vi "Named_Serial_Comms_orig.vi"(0 "Channel Name":string, 1 "Write String":string, 2 "Timeout/ms":u32=500, 4 "!Error retries":i32=10, 6 "!Timeout retries":i32=3, 9 "Port Name":string, 11 "Term Grep":string="\r$", 12 "Log Errors?":bool=TRUE, 13 "Terminate Count":i32) -> (3 "Read":string="This is simulation mode", 10 "millisecond timer value":u32, 14 "Timed out":bool, 15 "Serial Error":bool)   [LabVIEW 2010]
doc: "The Serial Communication VI performs bidirectional communication with a port. It initializes the port, writes a string to the port, and performs a read with timeout. The Read with Timeout will wait until a terminating character is received or the time limit is up, whichever comes first.\nThe initialisation parameters, terminating character, and timeout, are all set in the Serial Setup Global."
uses:
  Port_Params.ctl
  <vilib>/Instr/serial.llb/serpConfig.vi
panel:
  out "Buffer Trash":string
  out "Check Loops":i32
  out "Time Start":u32
  out "byte count":u32
  out "Terminated?":bool
  out "Case":string="Simulate"
  out "!Error retries remaining":i32=10
  out "length":i32
  out "Read chunks":string[](array[string])
  in  "Force setup reload":bool
  out "Port Initialised?":bool[](array[boolean])
  out "load setups error":bool
  out "Setting Number":i32
  in  "Error Description":string
  out "Read Loops":i32
  out "Audit trail":string[](array[string])=["Start", "Simulate"]
  in  "Save Setups?":bool
  out "Close Port error":i32
  out "read error code":i32
  out "n-bytes error code":i32
  out "Ports having file settings":string[](array[string])
  in  "Uppercase?":bool
  in  "Append Return?":bool
  out "Write error":i32
  in  "!stop":bool
  out "Port Initialisation Parameters":T1={"Name"="", "flow control etc."={"input XON/XOFF"=FALSE, "input HW Handshake"=FALSE, "input alt HW HShk"=FALSE, "output XON/XOFF"=FALSE, "output HW Handshake"=FALSE, "output alt HW HShk"=FALSE, "XOFF byte "=0, "XON byte"=0, "parity err byte"=0}, "buffer size"=0, "baud rate"=9600, "data bits"=8, "stop bits"=enum."1 bit", "parity"=enum."no parity"} {"flow control etc."."parity err byte" format="%.0x"; "flow control etc."."XON byte" format="%.0x"; "flow control etc."."XOFF byte" format="%.0x"; "data bits" min=5 max=8 step=1}
  out "Port Number":i32
  out "Initialise error":i32
  out "enumerated ports":string[](array[string])
  in  "Port Settings Array":T1[](array[typedef]) {"flow control etc."."parity err byte" format="%.0x"; "flow control etc."."XON byte" format="%.0x"; "flow control etc."."XOFF byte" format="%.0x"; "data bits" min=5 max=8 step=1}
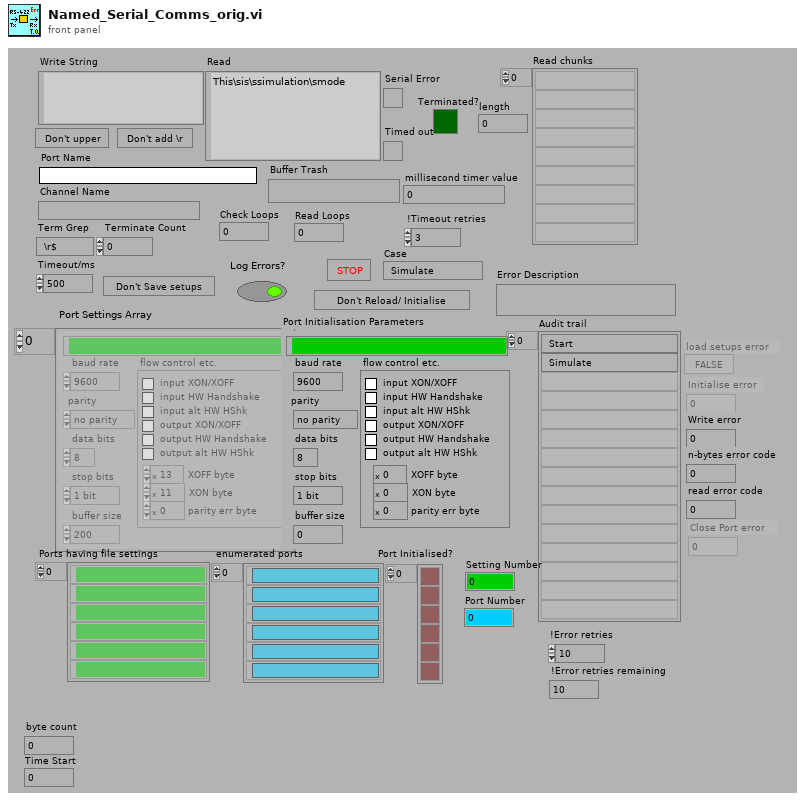
[diagram p1: front panel]
types:
  T1 = typedef "Port_Params.ctl" = cluster{"Name":string, "flow control etc.":cluster{"input XON/XOFF":bool, "input HW Handshake":bool, "input alt HW HShk":bool, "output XON/XOFF":bool, "output HW Handshake":bool, "output alt HW HShk":bool, "XOFF byte ":u8, "XON byte":u8, "parity err byte":u16}, "buffer size":u16, "baud rate":u32, "data bits":u16, "stop bits":enum16{"1 bit", "1.5 bits", "2 bits"}, "parity":enum16{"no parity", "odd parity", "even parity", "mark parity", "space parity"}}
  T2 = cluster{"input XON/XOFF":bool, "input HW Handshake":bool, "input alt HW HShk":bool, "output XON/XOFF":bool, "output HW Handshake":bool, "output alt HW HShk":bool, "XOFF byte ":u8, "XON byte":u8, "parity err byte":u16}
  T3 = enum16{"no parity", "odd parity", "even parity", "mark parity", "space parity"}
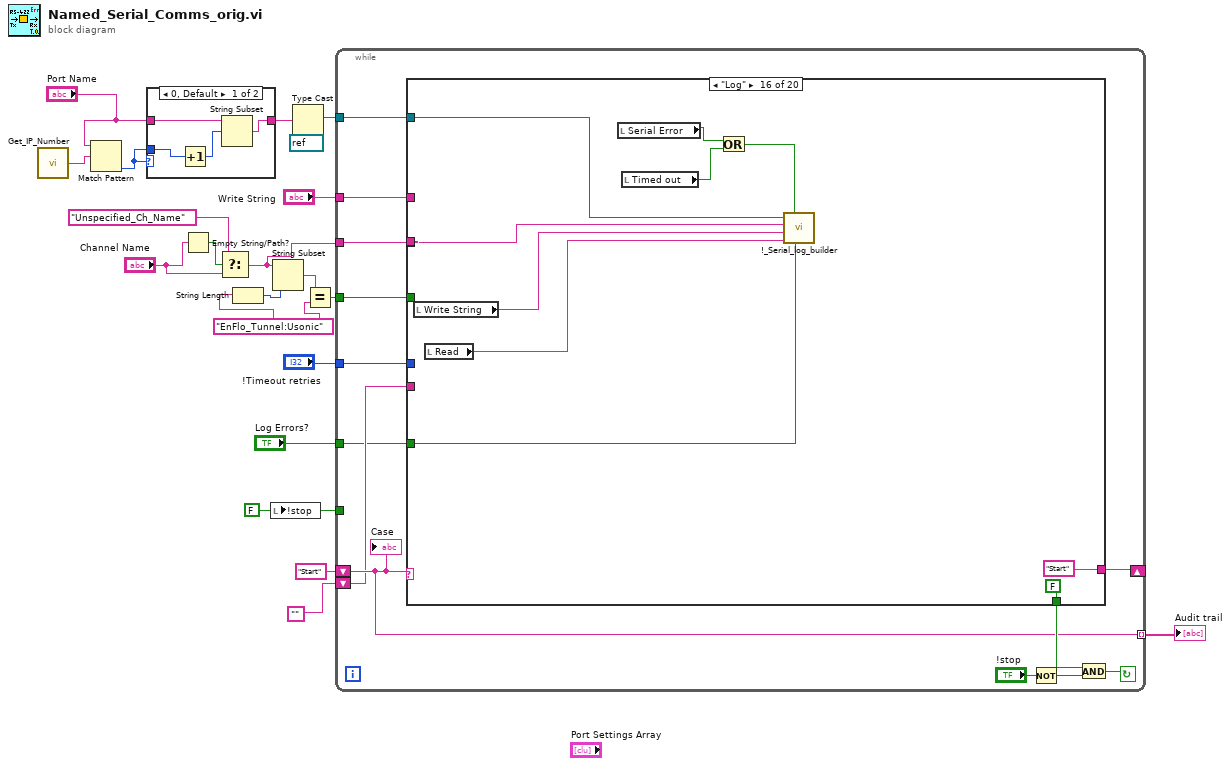
[diagram p0: block diagram]
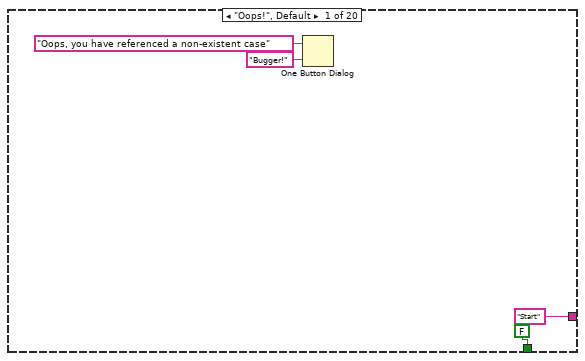
[diagram p3: hidden frame]
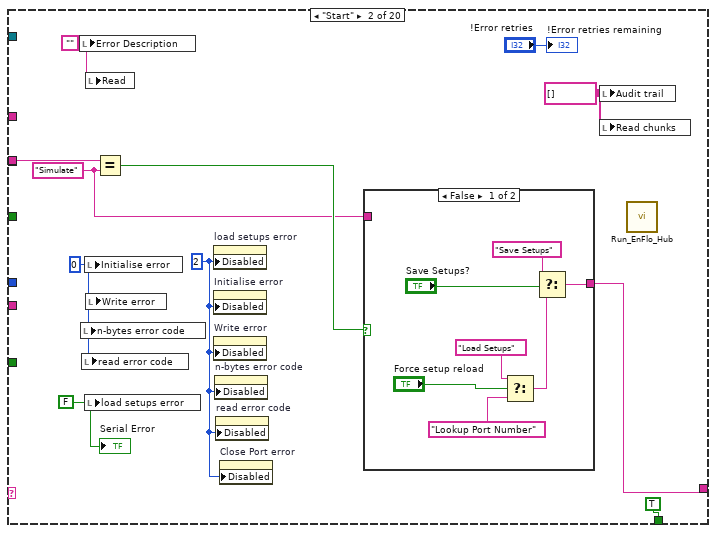
[diagram p4: hidden frame]
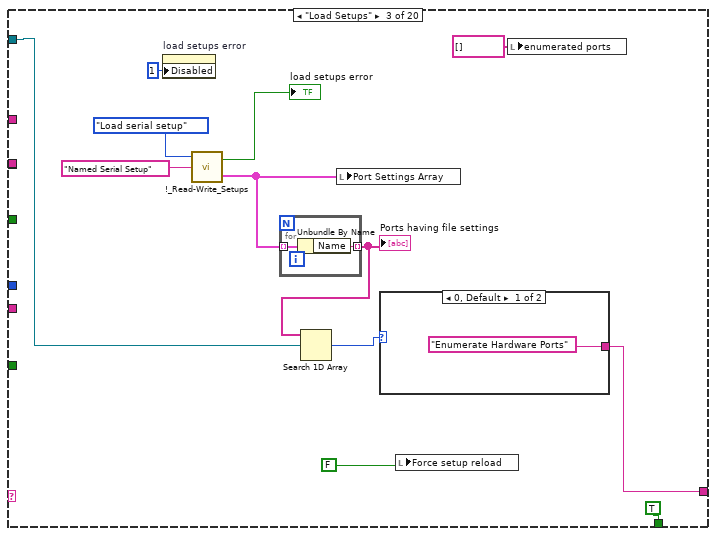
[diagram p6: hidden frame]
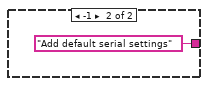
[diagram p7: hidden frame]
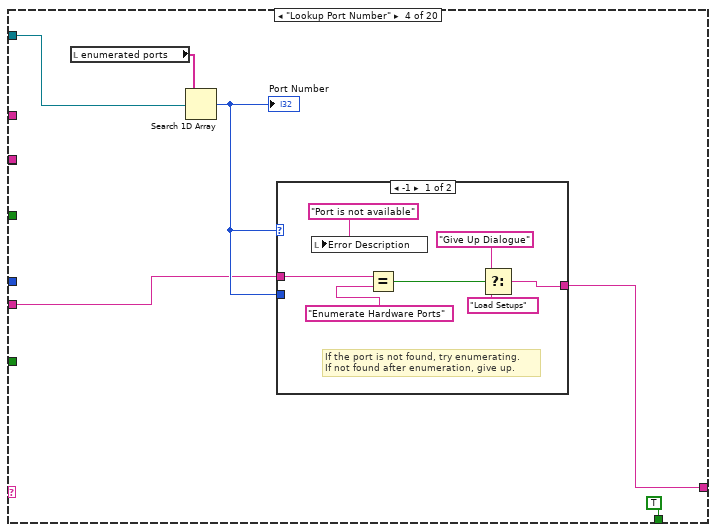
[diagram p8: hidden frame]
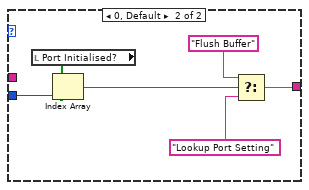
[diagram p9: hidden frame]
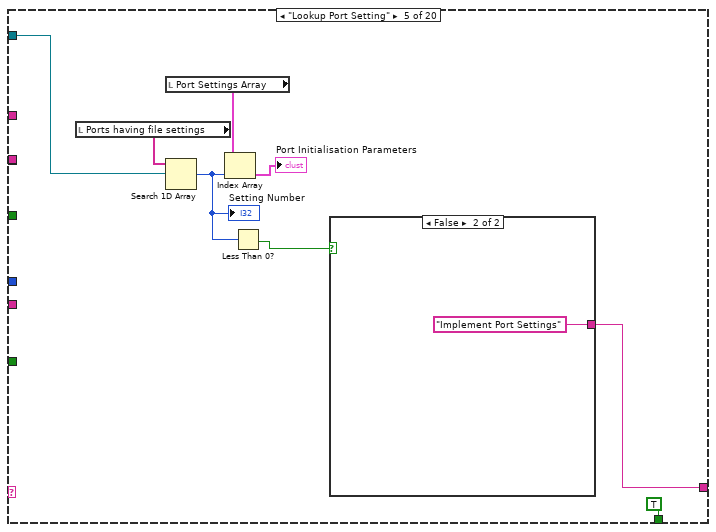
[diagram p10: hidden frame]
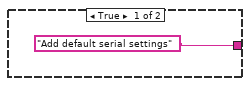
[diagram p11: hidden frame]
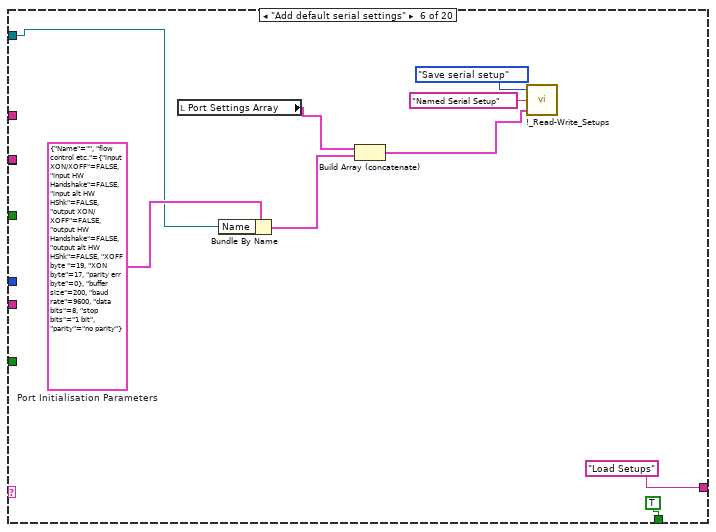
[diagram p12: hidden frame]
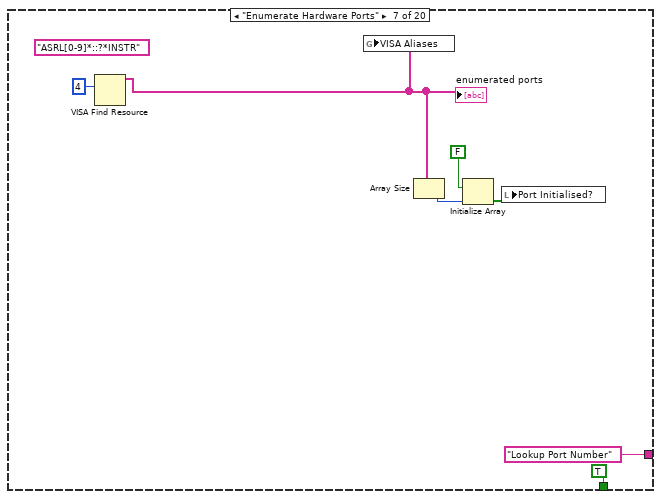
[diagram p13: hidden frame]
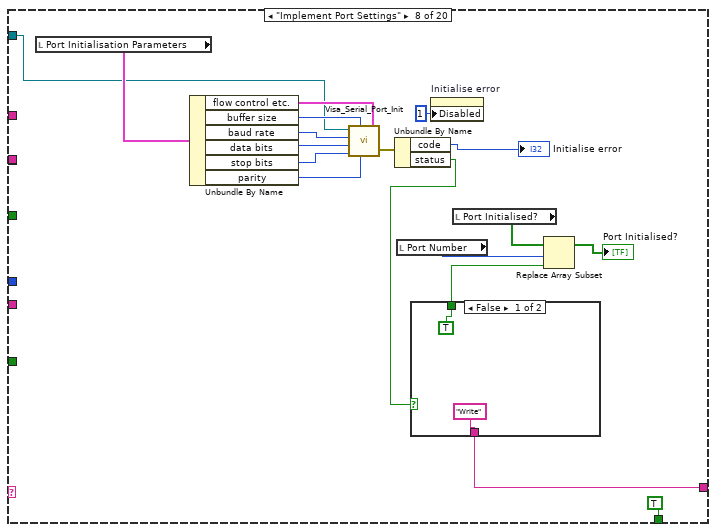
[diagram p14: hidden frame]
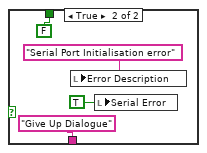
[diagram p15: hidden frame]
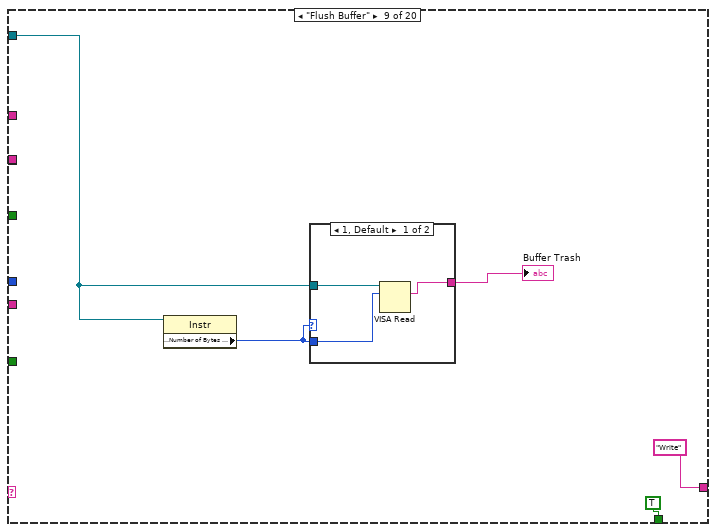
[diagram p16: hidden frame]
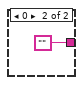
[diagram p17: hidden frame]
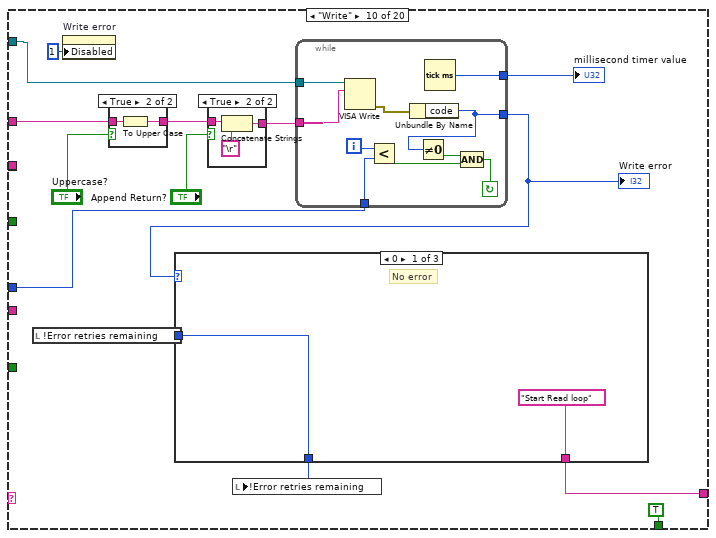
[diagram p18: hidden frame]
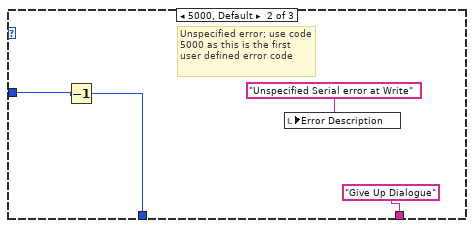
[diagram p19: hidden frame]
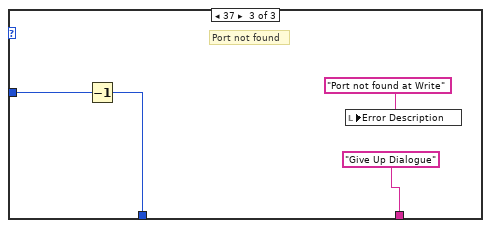
[diagram p20: hidden frame]
diagram:
  w13 = "EnFlo_Tunnel:Usonic"
  w19 = FALSE ("!stop")
  n1 = call "Get_IP_Number.vi"() -> ("IP Number"=w8:string)
  n2 = Match Pattern(string="Port Name", regular expression=w8) -> (offset past match=w9:i32)  [unwired: 1 in, 3 out]
  n3 = case shown="0, Default" w9 {
    tunnel: [w22 w26] -> w6
    tunnel: "Port Name" -> [w23 w26]
    tunnel: w9 -> [w25 _]
    frame 0, Default {
      n4 = Increment(x=w25) -> (x+1=w24:i32)
      n5 = String Subset(string=w23, offset (0)=w24) -> (substring=w22:string)  [unwired: 1 in]
    }
    frame -1 {
    }
  }
  n6 = Empty String/Path?(string/path="Channel Name") -> (empty?=w4:bool)
  n7 = Select(t="Unspecified_Ch_Name", s=w4, f="Channel Name") -> (s? t:f=w3:string)
  n8 = String Length(string=w13) -> (length=w15:i32)
  n9 = local write "!stop"(w19) -> ()
  n10 = String Subset(string=w3, length (rest)=w15) -> (substring=w14:string)  [unwired: 1 in]
  n11 = Type Cast(type=refnum<visa-resource-name> refnum ("dup VISA resource name"), x=w6) -> (*(type *) &x=w11:refnum<visa-resource-name>)
  n12 = Equal?(x=w14, y=w13) -> (x = y?=w12:bool)
  n13 = while {
    tunnel: "!Timeout retries" -> [w29]
    tunnel: w3 -> [w31]
    shift-left: "" -> [w30]
    tunnel: [w32] -> w18 mode=indexing
    tunnel: w19 -> [_]
    shift-left: "Start" -> [w32]
    shift-right: [w33] -> _
    tunnel: "Write String" -> [w38]
    tunnel: w11 -> [w39]
    tunnel: w12 -> [w28]
    tunnel: "Log Errors?" -> [w27]
    stop <- w36 continue-if-true
    n14 = case shown="\"Log\"" w32 {
      tunnel: w39 -> [_ _ w64 w84 w104 w113 _ w127 w148 w157 _ w208 w236 _ _ w300 w310 _ w332 _]
      tunnel: w38 -> [_ _ _ _ _ _ _ _ _ w166 _ _ _ _ _ _ w313 _ _ _]
      tunnel: ["Start" ("f") w54 w67 w81 w100 "Load Setups" ("f") "Lookup Port Number" w132 "Write" ("f") w162 "Bytes At Serial Port?" ("f") w213 w250 w265 w295 "Start" "Start" "Start" "Start" ("f") "Load Setups" ("f")] -> w33
      tunnel: [FALSE TRUE TRUE TRUE TRUE TRUE TRUE TRUE TRUE TRUE TRUE TRUE TRUE TRUE TRUE FALSE FALSE TRUE FALSE TRUE] -> w37
      tunnel: w31 -> [_ w47 _ _ _ _ _ _ _ _ _ _ _ _ _ w306 _ _ _ _]
      tunnel: w31 -> [_ _ _ _ _ _ _ _ _ _ _ _ _ _ _ _ w311 _ _ _]
      tunnel: w30 -> [_ _ _ w79 _ _ _ _ _ _ _ _ _ _ _ _ _ _ _ _]
      tunnel: w29 -> [_ _ _ _ _ _ _ _ _ w158 _ w210 _ _ _ _ _ _ _ _]
      tunnel: w28 -> [_ _ _ _ _ _ _ _ _ _ _ _ w240 _ _ _ _ _ _ _]
      tunnel: w27 -> [_ _ _ _ _ _ _ _ _ _ _ _ _ _ _ w299 _ _ _ _]
      frame "Oops!", Default {
        n15 = One Button Dialog(message="Oops, you have referenced a non-existent case", button name ("OK")="Bugger!") -> ()  [unwired: 1 out]
      }
      frame "Start" {
        w44 = string[] [] ("Audit trail")
        w45 = "Simulate" ("y")
        w51 = 0 ("Initialise error")
        w49 = FALSE
        w50 = u8 2 ("Write Attribute")
        w52 = ""
        n16 = local write "Error Description"(w52) -> ()
        n17 = local write "n-bytes error code"(w51) -> ()
        n18 = local write "read error code"(w51) -> ()
        n19 = local write "Initialise error"(w51) -> ()
        n20 = local write "load setups error"(w49) -> ()
        n21 = local write "Read"(w52) -> ()
        n22 = local write "Write error"(w51) -> ()
        n23 = Equal?(x=w47, y=w45) -> (x = y?=w46:bool)
        n24 = property on="load setups error" class="Bool (strict)"("Disabled"=w50) -> ()  [unwired: 2 in, 2 out]
        n25 = property on="Initialise error" class="DigNum (strict)"("Disabled"=w50) -> ()  [unwired: 2 in, 2 out]
        n26 = property on="Write error" class="DigNum (strict)"("Disabled"=w50) -> ()  [unwired: 2 in, 2 out]
        n27 = property on="n-bytes error code" class="DigNum (strict)"("Disabled"=w50) -> ()  [unwired: 2 in, 2 out]
        n28 = property on="read error code" class="DigNum (strict)"("Disabled"=w50) -> ()  [unwired: 2 in, 2 out]
        n29 = property on="Close Port error" class="DigNum (strict)"("Disabled"=w50) -> ()  [unwired: 2 in, 2 out]
        n30 = case shown="False" w46 {
          tunnel: [w57 w62] -> w54
          tunnel: w45 -> [_ w62]
          frame False {
            n31 = Select(t="Load Setups" ("f"), s="Force setup reload", f="Lookup Port Number") -> (s? t:f=w58:string)
            n32 = Select(t="Save Setups", s="Save Setups?", f=w58) -> (s? t:f=w57:string)
          }
          frame True {
          }
        }
        n33 = local write "Audit trail"(w44) -> ()
        n34 = local write "Read chunks"(w44) -> ()
        n35 = call "Run_EnFlo_Hub.vi"() -> ()  [unwired: 8 in]
        "Serial Error" <- w49
        "!Error retries remaining" <- "!Error retries"
      }
      frame "Load Setups" {
        n36 = property on="load setups error" class="Bool (strict)"("Disabled"=u8 1 ("Write Attribute")) -> ()  [unwired: 2 in, 2 out]
        n37 = call "!_Read-Write_Setups.vi"("Setup Name"="Named Serial Setup", "Mode"=enum16{"Load serial setup", "Save serial setup"}."Load serial setup") -> ("Port Settings Array Out"=w68:T1[], "error unflattening"=→"load setups error":bool)  [unwired: 1 in]
        n38 = for {
          tunnel: w68 -> [w78] mode=indexing
          tunnel: [w77] -> w65 mode=indexing
          n39 = Unbundle By Name(w78) -> ("Name"=w77:string)
        }
        "Ports having file settings" <- w65
        n40 = Search 1D Array(1D array=w65, element=w64) -> (index of element=w63:i32)  [unwired: 1 in]
        n41 = local write "Port Settings Array"(w68) -> ()
        n42 = case shown="0, Default" w63 {
          tunnel: ["Enumerate Hardware Ports" "Add default serial settings"] -> w67
          frame 0, Default {
          }
          frame -1 {
          }
        }
        n43 = local write "Force setup reload"(FALSE ("Force setup reload")) -> ()
        n44 = local write "enumerated ports"(string[] [] ("enumerated ports")) -> ()
      }
      frame "Lookup Port Number" {
        n45 = local read "enumerated ports"() -> (w83:string[])
        n46 = Search 1D Array(1D array=w83, element=w84) -> (index of element=w80:i32)  [unwired: 1 in]
        "Port Number" <- w80
        n47 = case shown="-1" w80 {
          tunnel: [w91 w97] -> w81
          tunnel: w80 -> [_ w95]
          tunnel: w79 -> [w88 _]
          frame -1 {
            # "If the port is not found, try enumerating.\nIf not found after enumeration, give up."
            n48 = local write "Error Description"("Port is not available" ("Error Description")) -> ()
            n49 = Equal?(x=w88, y="Enumerate Hardware Ports" ("f")) -> (x = y?=w90:bool)
            n50 = Select(t="Give Up Dialogue" ("f"), s=w90, f="Load Setups") -> (s? t:f=w91:string)
          }
          frame 0, Default {
            n51 = local read "Port Initialised?"() -> (w96:bool[])
            n52 = Index Array(array=w96, index=w95) -> (element=w94:bool)
            n53 = Select(t="Flush Buffer" ("f"), s=w94, f="Lookup Port Setting") -> (s? t:f=w97:string)
          }
        }
      }
      frame "Lookup Port Setting" {
        n54 = local read "Ports having file settings"() -> (w105:string[])
        n55 = local read "Port Settings Array"() -> (w102:T1[])
        n56 = Search 1D Array(1D array=w105, element=w104) -> (index of element=w99:i32)  [unwired: 1 in]
        "Setting Number" <- w99
        n57 = Index Array(array=w102, index=w99) -> (element=→"Port Initialisation Parameters":T1)
        n58 = Less Than 0?(x=w99) -> (x < 0?=w98:bool)
        n59 = case shown="False" w98 {
          tunnel: ["Add default serial settings" "Implement Port Settings"] -> w100
          frame True {
          }
          frame False {
          }
        }
      }
      frame "Add default serial settings" {
        w115 = T1 {"Name"="", "flow control etc."={"input XON/XOFF"=FALSE, "input HW Handshake"=FALSE, "input alt HW HShk"=FALSE, "output XON/XOFF"=FALSE, "output HW Handshake"=FALSE, "output alt HW HShk"=FALSE, "XOFF byte "=19, "XON byte"=17, "parity err byte"=0}, "buffer size"=200, "baud rate"=9600, "data bits"=8, "stop bits"=enum."1 bit", "parity"=enum."no parity"}  # Port Initialisation Parameters
        n60 = local read "Port Settings Array"() -> (w116:T1[])
        n61 = Bundle By Name(cluster=w115, "Name"=w113) -> (w114:T1)
        n62 = Build Array (concatenate)(w116, w114) -> (w110:T1[])
        n63 = call "!_Read-Write_Setups.vi"("Port Settings Array In"=w110, "Setup Name"="Named Serial Setup", "Mode"=enum16{"Load serial setup", "Save serial setup"}."Save serial setup") -> ()  [unwired: 2 out]
      }
      frame "Enumerate Hardware Ports" {
        (unwired) "ASRL[0-9]*::?*INSTR" ("expression (\"?*\")")
        n64 = VISA Find Resource(10:u32 4 ("search mode (0)")) -> (3:w118:string[])  [unwired: 2 in, 2 out]
        "enumerated ports" <- w118
        n65 = global write "serpConfig.vi" "VISA Aliases"(w118) -> ()
        n66 = Array Size(array=w118) -> (size(s)=w121:i32)
        n67 = Initialize Array(FALSE, w121) -> (w120:bool[])
        n68 = local write "Port Initialised?"(w120) -> ()
      }
      frame "Implement Port Settings" {
        n69 = local read "Port Initialisation Parameters"() -> (w135:T1)
        n70 = Unbundle By Name(w135) -> ("flow control etc."=w141:T2, "buffer size"=w140:u16, "baud rate"=w139:u32, "data bits"=w138:u16, "stop bits"=w137:enum16{"1 bit", "1.5 bits", "2 bits"}, "parity"=w136:T3)
        n71 = call "Visa_Serial_Port_Init.vi"("flow control etc."=w141, "parity"=w136, "buffer size"=w140, "stop bits"=w137, "data bits"=w138, "baud rate"=w139, "Visa Port Name"=w127) -> ("error out"=w126:errorcluster)
        n72 = Unbundle By Name(w126) -> ("code"=→"Initialise error":i32, "status"=w124:bool)
        n73 = local read "Port Number"() -> (w129:i32)
        n74 = case shown="False" w124 {
          tunnel: ["Write" "Give Up Dialogue"] -> w132
          tunnel: [TRUE ("Element Data") FALSE ("Element Data")] -> w128
          frame False {
          }
          frame True {
            n75 = local write "Error Description"("Serial Port Initialisation error" ("Error Description")) -> ()
            n76 = local write "Serial Error"(TRUE ("Serial Error")) -> ()
          }
        }
        n77 = property on="Initialise error" class="DigNum (strict)"("Disabled"=u8 1 ("Write Attribute")) -> ()  [unwired: 2 in, 2 out]
        n78 = local read "Port Initialised?"() -> (w130:bool[])
        n79 = Replace Array Subset(array=w130, new element=w128, index=w129) -> (→"Port Initialised?":bool[])
      }
      frame "Flush Buffer" {
        n80 = property class="Instr"(reference=w148) -> ("Serial Settings:Number of Bytes at Serial Port"=w149:u32)  [unwired: 1 in, 2 out]
        n81 = case shown="1, Default" w149 {
          tunnel: [w155 ""] -> w151
          tunnel: w148 -> [w154 _]
          tunnel: w149 -> [w153 _]
          frame 1, Default {
            n82 = VISA Read(VISA resource name=w154, byte count=w153) -> (read buffer=w155:string)  [unwired: 1 in, 3 out]
          }
          frame 0 {
          }
        }
        "Buffer Trash" <- w151
      }
      frame "Write" {
        n83 = local read "!Error retries remaining"() -> (w160:i32)
        n84 = property on="Write error" class="DigNum (strict)"("Disabled"=u8 1 ("Write Attribute")) -> ()  [unwired: 2 in, 2 out]
        n85 = case shown="True" "Uppercase?" {
          tunnel: w166 -> [w195 w197]
          tunnel: [w195 w196] -> w168
          frame False {
          }
          frame True {
            n86 = To Upper Case(1:w197) -> (0:w196:string)
          }
        }
        n87 = case shown="True" "Append Return?" {
          tunnel: w168 -> [w191 w194]
          tunnel: [w191 w193] -> w165
          frame False {
          }
          frame True {
            n88 = Concatenate Strings(w194, "\r") -> (w193:string)
          }
        }
        n89 = while {
          tunnel: w158 -> [w175]
          tunnel: [w174] -> w161
          tunnel: w165 -> [w171]
          tunnel: [w180] -> w170
          tunnel: w157 -> [w172]
          i -> [w179]
          stop <- w176 continue-if-true
          n90 = VISA Write(VISA resource name=w172, write buffer=w171) -> (error out=w173:errorcluster)  [unwired: 1 in, 2 out]
          n91 = Less?(x=w179, y=w175) -> (x < y?=w178:bool)
          n92 = Unbundle By Name(w173) -> ("code"=w174:i32)
          n93 = Not Equal To 0?(x=w174) -> (x != 0?=w177:bool)
          n94 = Tick Count (ms)() -> (millisecond timer value=w180:u32)
          n95 = Compound Arithmetic op=AND(w177, w178) -> (w176:bool)
        }
        "Write error" <- w161
        "millisecond timer value" <- w170
        n96 = case shown="0" w161 {
          tunnel: ["Start Read loop" "Give Up Dialogue" "Give Up Dialogue"] -> w162
          tunnel: w160 -> [w181 w184 w188]
          tunnel: [w181 w183 w187] -> w159
          frame 0 {
            # "No error"
          }
          frame 5000, Default {
            # "Unspecified error; use code 5000 as this is the first user defined error code"
            n97 = Decrement(x=w184) -> (x-1=w183:i32)
            n98 = local write "Error Description"("Unspecified Serial error at Write" ("Error Description")) -> ()
          }
          frame 37 {
            # "Port not found"
            n99 = Decrement(x=w188) -> (x-1=w187:i32)
            n100 = local write "Error Description"("Port not found at Write" ("Error Description")) -> ()
          }
        }
        n101 = local write "!Error retries remaining"(w159) -> ()
      }
      frame "Start Read loop" {
        w198 = FALSE ("Timed out")
        n102 = Tick Count (ms)() -> (millisecond timer value=→"Time Start":u32)
        n103 = local write "Read chunks"(string[] [] ("Read chunks")) -> ()
        n104 = local write "Read Loops"(0 ("Read Loops")) -> ()
        n105 = local write "Timed out"(w198) -> ()
        n106 = local write "Terminated?"(w198) -> ()
        n107 = local write "Check Loops"(0 ("Check Bytes Loops")) -> ()
        n108 = local write "Read"("") -> ()
        n109 = property on="n-bytes error code" class="DigNum (strict)"("Disabled"=u8 1 ("Write Attribute")) -> ()  [unwired: 2 in, 2 out]
        n110 = property on="read error code" class="DigNum (strict)"("Disabled"=u8 1 ("Write Attribute")) -> ()  [unwired: 2 in, 2 out]
      }
      frame "Bytes At Serial Port?" {
        n111 = while {
          tunnel: w210 -> [w222]
          tunnel: [w221] -> w209
          tunnel: [w223] -> w216
          tunnel: w208 -> [w218]
          i -> [w226]
          stop <- w224 continue-if-true
          n112 = property class="Instr"(reference=w218) -> (error out=w220:errorcluster, "Serial Settings:Number of Bytes at Serial Port"=w221:u32)  [unwired: 1 in, 1 out]
          "byte count" <- w221
          n113 = Unbundle By Name(w220) -> ("code"=w219:i32)
          "n-bytes error code" <- w219
          n114 = Less?(x=w226, y=w222) -> (x < y?=w225:bool)
          n115 = Equal To 0?(x=w219) -> (x = 0?=w223:bool)
          n116 = Compound Arithmetic op=AND(invert w223, w225) -> (w224:bool)
          n117 = case shown="True" w224 {
            frame False {
            }
            frame True {
              n118 = Wait (ms)(milliseconds to wait=u32 5) -> ()  [unwired: 1 out]
            }
          }
        }
        n119 = local read "Check Loops"() -> (w212:i32)
        n120 = case shown="1, Default" w209 {
          tunnel: ["Serial Port Read" ("f") "Check for Termination" ("f")] -> w214
          frame 1, Default {
          }
          frame 0 {
            n121 = Wait (ms)(milliseconds to wait=u32 1) -> ()  [unwired: 1 out]
          }
        }
        n122 = Increment(x=w212) -> (x+1=→"Check Loops":i32)
        n123 = Select(t=w214, s=w216, f="Log") -> (s? t:f=w213:string)
      }
      frame "Serial Port Read" {
        n124 = local read "byte count"() -> (w238:u32)
        n125 = Greater?(x=w238, y=u32 1) -> (0:w239:bool)
        n126 = And(x=w239, y=w240) -> (x .and. y?=w237:bool)
        n127 = case shown="True" w237 {
          tunnel: w238 -> [w256 w258]
          tunnel: [w256 w257] -> w235
          frame False {
          }
          frame True {
            n128 = Decrement(x=w258) -> (x-1=w257:u32)
          }
        }
        n129 = VISA Read(VISA resource name=w236, byte count=w235) -> (read buffer=w233:string, error out=w234:errorcluster)  [unwired: 1 in, 2 out]
        n130 = local read "Read"() -> (w253:string)
        n131 = Unbundle By Name(w234) -> ("code"=w232:i32)
        n132 = case shown="0, Default" w232 {
          selector: w232 -> [w254 _]
          tunnel: [w254 0 ("code")] -> w231
          frame 0, Default {
          }
          frame 1073676294 {
          }
        }
        "read error code" <- w231
        n133 = Concatenate Strings(w253, w233) -> (w244:string)
        "Read" <- w244
        n134 = local read "Read chunks"() -> (w247:string[])
        n135 = Equal To 0?(x=w231) -> (x = 0?=w249:bool)
        n136 = local read "Read Loops"() -> (w243:i32)
        n137 = Build Array (concatenate)(w247, w233) -> (→"Read chunks":string[])
        n138 = String Length(string=w244) -> (length=→"length":i32)
        n139 = Increment(x=w243) -> (x+1=→"Read Loops":i32)
        n140 = Select(t="Check for Termination" ("f"), s=w249, f="Log") -> (s? t:f=w250:string)
      }
      frame "Check for Termination" {
        n141 = local read "Read"() -> (w267:string)
        n142 = Empty String/Path?(string/path="Term Grep") -> (empty?=w268:bool)
        n143 = case shown="False" w268 {
          tunnel: "Terminate Count" -> [w272 w287]
          tunnel: w267 -> [w274 w288]
          tunnel: [w269 w286] -> w262
          tunnel: "Term Grep" -> [w275 _]
          frame False {
            n144 = Decrement(x=w272) -> (x-1=w271:i32)
            n145 = while {
              tunnel: [w276] -> w270
              tunnel: w271 -> [w279]
              shift-left: 0 -> [w283]
              shift-right: [w282] -> _
              tunnel: w274 -> [w284]
              tunnel: w275 -> [w285]
              i -> [w280]
              stop <- w277 continue-if-true
              n146 = Match Pattern(string=w284, regular expression=w285, offset (0)=w283) -> (match substring=w276:string, offset past match=w282:i32)  [unwired: 2 out]
              n147 = Less?(x=w280, y=w279) -> (x < y?=w278:bool)
              n148 = Greater Or Equal To 0?(x=w282) -> (x >= 0?=w281:bool)
              n149 = Compound Arithmetic op=AND(w281, w278) -> (w277:bool)
            }
            n150 = Empty String/Path?(string/path=w270) -> (empty?=w269:bool)
          }
          frame True {
            n151 = String Length(string=w288) -> (length=w289:i32)
            n152 = Less?(x=w289, y=w287) -> (x < y?=w286:bool)
          }
        }
        n153 = Not(x=w262) -> (.not. x?=w259:bool)
        "Terminated?" <- w259
        n154 = Select(t="Log" ("f"), s=w259, f="TimeOut?") -> (s? t:f=w265:string)
      }
      frame "TimeOut?" {
        n155 = local read "Time Start"() -> (w296:u32)
        n156 = Tick Count (ms)() -> (millisecond timer value=w297:u32)
        n157 = Subtract(x=w297, y=w296) -> (x-y=w298:u32)
        n158 = Greater?(x=w298, y="Timeout/ms") -> (0:w291:bool)
        "Timed out" <- w291
        n159 = Select(t="Log" ("f"), s=w291, f="Bytes At Serial Port?") -> (s? t:f=w295:string)
      }
      frame "Log" {
        n160 = local read "Write String"() -> (w305:string)
        n161 = local read "Read"() -> (w304:string)
        n162 = local read "Serial Error"() -> (w303:bool)
        n163 = local read "Timed out"() -> (w301:bool)
        n164 = Or(x=w303, y=w301) -> (x .or. y?=w302:bool)
        n165 = call "!_Serial_log_builder.vi"("Port Name"=w300, "Comms Error"=w302, "Channel Name"=w306, "Write String"=w305, "Log Errors?"=w299, "Read"=w304) -> ()  [unwired: 3 in]
      }
      frame "Give Up Dialogue" {
        w321 = FALSE  # Dialog Box
        n166 = Format Into String(format string="%s%s%s%s%s%s\" ", initial string="Error Description", " whilst trying to write \n\"", w313, "\" to Channel \"", w311, "\" at Port \"" ("Input 5"), w310) -> (resulting string=w320:string)  [unwired: 1 in, 1 out]
        n167 = Bundle By Name(cluster=errorcluster {"status"=FALSE, "code"=0, "source"=""} ("error in (no error)"), "status"=TRUE ("Bundle Element"), "source"=w320) -> (w322:errorcluster)
        n168 = call "EnFlo_Error_Handler.vi"("error in (no error)"=w322, "Dialog Box (T)"=w321) -> ()  [unwired: 1 in, 3 out]
      }
      frame "Close All Ports" {
        n169 = local read "enumerated ports"() -> (w324:string[])
        n170 = for {
          tunnel: w324 -> [w328] mode=indexing
          n171 = VISA Close(VISA resource name=w328) -> (error out=w330:errorcluster)  [unwired: 1 in]
          n172 = Unbundle By Name(w330) -> ("code"=→"Close Port error":i32)
        }
        n173 = property on="Close Port error" class="DigNum (strict)"("Disabled"=u8 1 ("Write Attribute")) -> ()  [unwired: 2 in, 2 out]
      }
      frame "Simulate" {
        (unwired) "This is simulation mode" ("Read")
        n174 = Tick Count (ms)() -> (millisecond timer value=w331:u32)
        n175 = local write "millisecond timer value"(w331) -> ()
        n176 = local write "Read"(w332) -> ()
      }
      frame "Save Setups" {
        n177 = local read "Port Settings Array"() -> (w338:T1[])
        n178 = call "!_Read-Write_Setups.vi"("Port Settings Array In"=w338, "Setup Name"="Named Serial Setup", "Mode"=enum16{"Load serial setup", "Save serial setup"}."Save serial setup") -> ()  [unwired: 2 out]
      }
    }
    n179 = Not(x="!stop") -> (.not. x?=w34:bool)
    n180 = And(x=w37, y=w34) -> (x .and. y?=w36:bool)
    "Case" <- w32
  }
  "Audit trail" <- w18
